vi "Wiimote Open.vi"(8 "error in (no error)":errorcluster, 10 "Connect to all?":bool) -> (0 "error out":errorcluster, 2 "# Wiimotes connected":i32, 3 "LV WiiMote Interface":T1)   [LabVIEW 2012, in "LV Wiimote Interface.lvclass"]
uses:
  LV Wiimote Interface.lvclass
  Controls/LV Wiimote Interface.ctl
  C:/Program Files/National Instruments/LabVIEW 2012/vi.lib/LabVIEW Hacker/WiiMote/Dependencies/WiimoteLib.dll
  Program Files/National Instruments/LabVIEW 2012/vi.lib/LabVIEW Hacker/WiiMote/Dependencies/WiimoteLib.dll
  LV Wiimote Interface.lvclass/LV Wiimote Interface.ctl
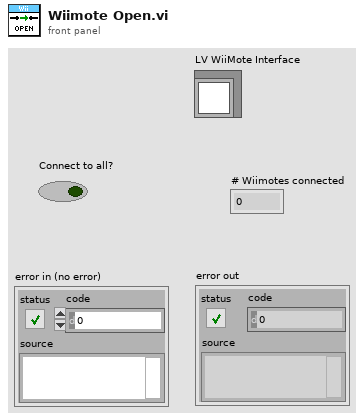
[diagram p1: front panel]
types:
  T1 = typedef "LV Wiimote Interface.ctl" = refnum<class "LV Wiimote Interface.lvclass">
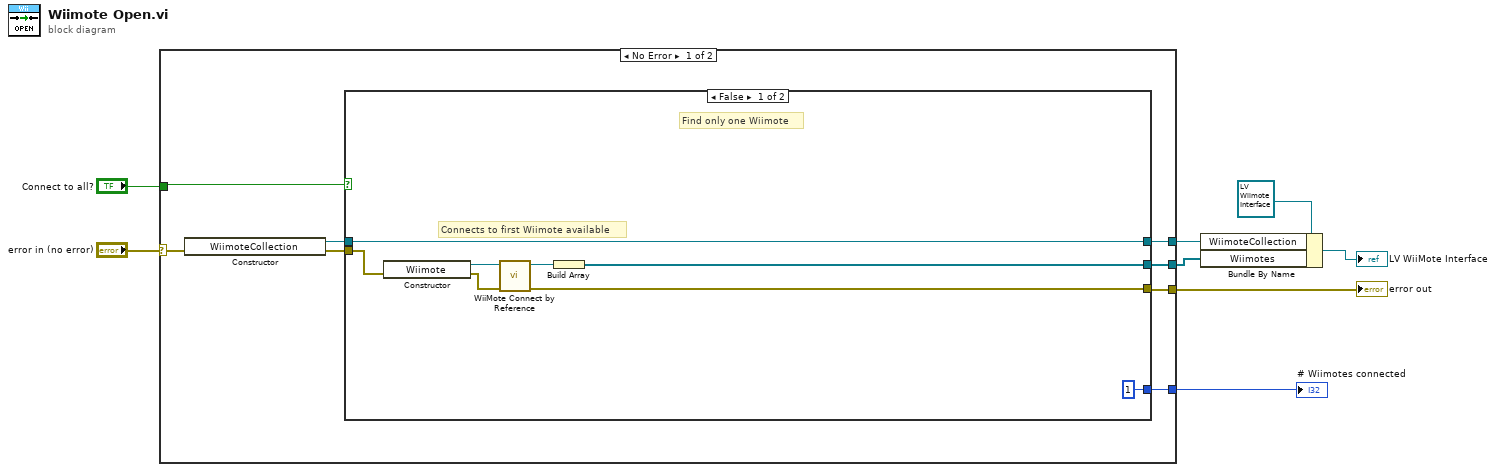
[diagram p0: block diagram]
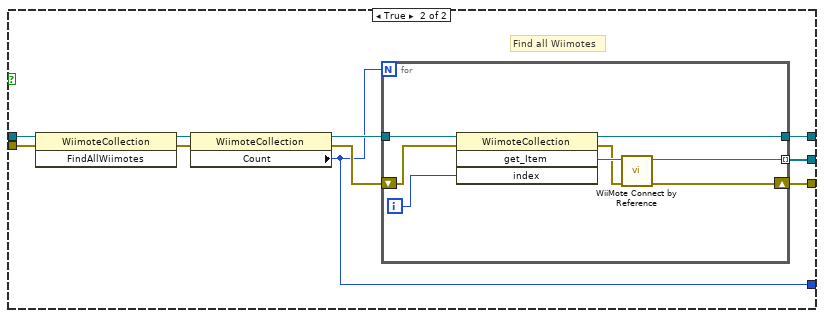
[diagram p2: hidden frame]
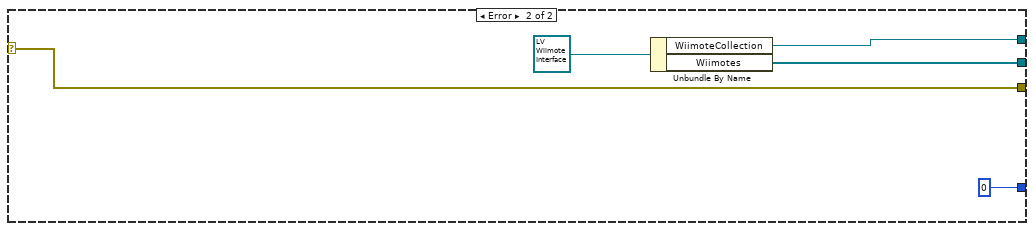
[diagram p3: hidden frame]
diagram:
  n1 = case shown="No Error" "error in (no error)" {
    selector: "error in (no error)" -> [w14 w47]
    tunnel: [w11 w47] -> w7
    tunnel: "Connect to all?" -> [w10 _]
    tunnel: [w13 w45] -> w3
    tunnel: [w12 w44] -> w2
    tunnel: [w9 0 ("Count")] -> w1
    frame No Error {
      n2 = constructor class="WiimoteCollection"(error in=w14) -> (reference out=w16:refnum<k24>, error out=w15:errorcluster)  [unwired: 2 in, 1 out]
      n3 = case shown="False" w10 {
        tunnel: w16 -> [w18 w34]
        tunnel: w15 -> [w24 w33]
        tunnel: [w18 w32] -> w13
        tunnel: [w19 w31] -> w12
        tunnel: [w20 w30] -> w11
        tunnel: [1 ("Count") w25] -> w9
        frame False {
          # "Connects to first Wiimote available"
          # "Find only one Wiimote"
          n4 = constructor class="Wiimote"(error in=w24) -> (reference out=w23:refnum<k24>, error out=w22:errorcluster)  [unwired: 2 in, 1 out]
          n5 = call "WiiMote Connect by Reference.vi"("error in (no error)"=w22, "WiiMote Reference"=w23) -> ("error out"=w20:errorcluster, "WiiMote Reference out"=w21:refnum<k24>)  [unwired: 8 in]
          n6 = Build Array(w21) -> (w19:refnum<k24>[])
        }
        frame True {
          # "Find all Wiimotes"
          n7 = invoke class="WiimoteCollection" method="FindAllWiimotes"(reference=w34, error in=w33) -> (reference out=w29:refnum<k24>, error out=w28:errorcluster)  [unwired: 1 in, 1 out]
          n8 = property class="WiimoteCollection"(reference=w29, error in=w28) -> (reference out=w27:refnum<k24>, error out=w26:errorcluster, "Count"=w25:i32)
          n9 = for {
            N: w25 -> [_]
            tunnel: [w41] -> w32
            tunnel: [w37] -> w31 mode=indexing
            shift-right: [w36] -> w30
            shift-left: w26 -> [w42]
            tunnel: w27 -> [w35]
            i -> [w39]
            n10 = invoke class="WiimoteCollection" method="get_Item"(reference=w35, error in=w42, "index"=w39) -> (reference out=w41:refnum<k24>, error out=w38:errorcluster, "get_Item"=w40:refnum<k24>)  [unwired: 1 in, 1 out]
            n11 = call "WiiMote Connect by Reference.vi"("error in (no error)"=w38, "WiiMote Reference"=w40) -> ("error out"=w36:errorcluster, "WiiMote Reference out"=w37:refnum<k24>)  [unwired: 8 in]
          }
        }
      }
    }
    frame Error {
      n12 = Unbundle By Name(T1 refnum ("LV WiiMote Interface 2")) -> ("WiimoteCollection"=w45:refnum<k24>, "Wiimotes"=w44:refnum<k24>[])
    }
  }
  "error out" <- w7
  "# Wiimotes connected" <- w1
  n13 = Bundle By Name(cluster=T1 refnum ("LV WiiMote Interface 2"), "WiimoteCollection"=w3, "Wiimotes"=w2) -> (→"LV WiiMote Interface":T1)
